vi "Dashboard Main.vi"() -> ()   [LabVIEW 2015]
uses:
  Custom Code/General/RemoteFiles/connectionData.ctl
panel:
  in  "stopButton":bool
  in  "MainDashTab":T1(tab)
  out "Robot IP":string
  in  "Window Docked?":bool
  in  "MainConfigCommunicationData":T3
  out "TeleopImageDisplay":T4(plugin-control)
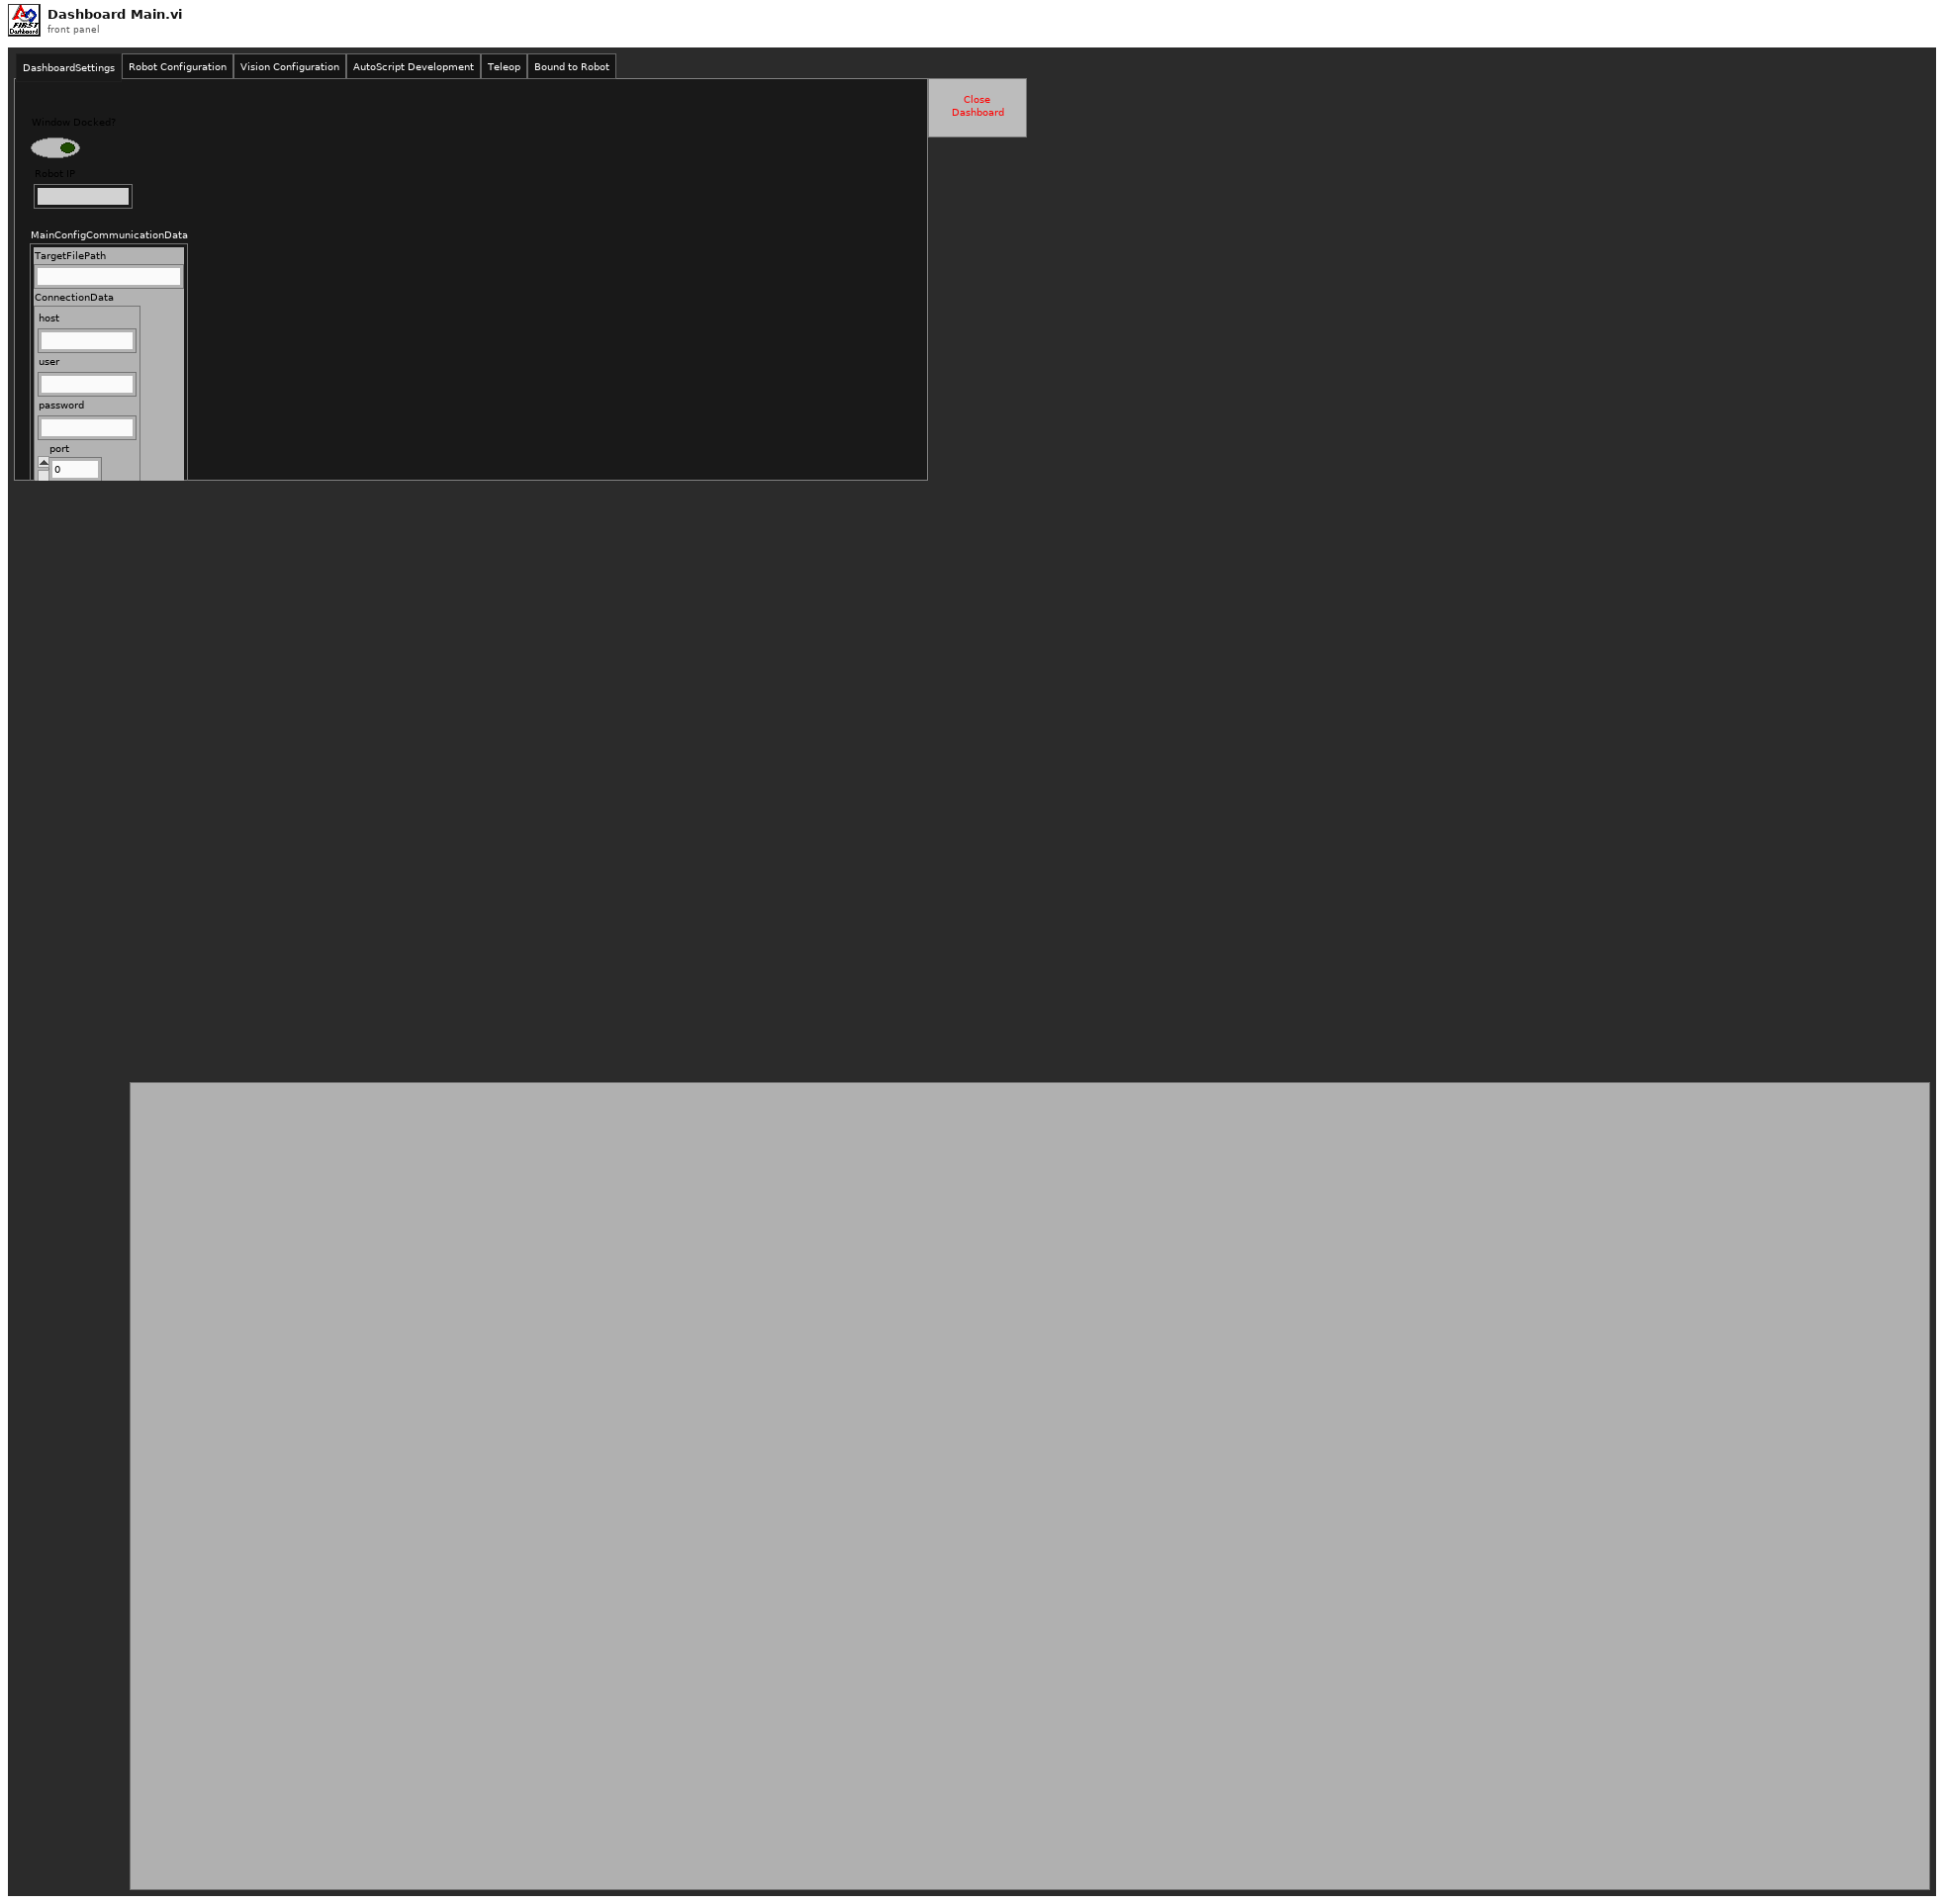
[diagram p1: front panel]
types:
  T1 = enum32{"DashboardSettings", "Robot Configuration", "Vision Configuration", "AutoScript Development", "Teleop", "Bound to Robot"}
  T2 = typedef "connectionData.ctl" = cluster{"host":string, "user":string, "password":string, "port":u16}
  T3 = cluster{"TargetFilePath":string, "ConnectionData":T2}
  T4 = typedef "IMAQ Image.ctl" = refnum<image>
  T5 = cluster{"notifier out":refnum<notifier>, "notifier out":refnum<notifier>, "notifier out":refnum<notifier>}
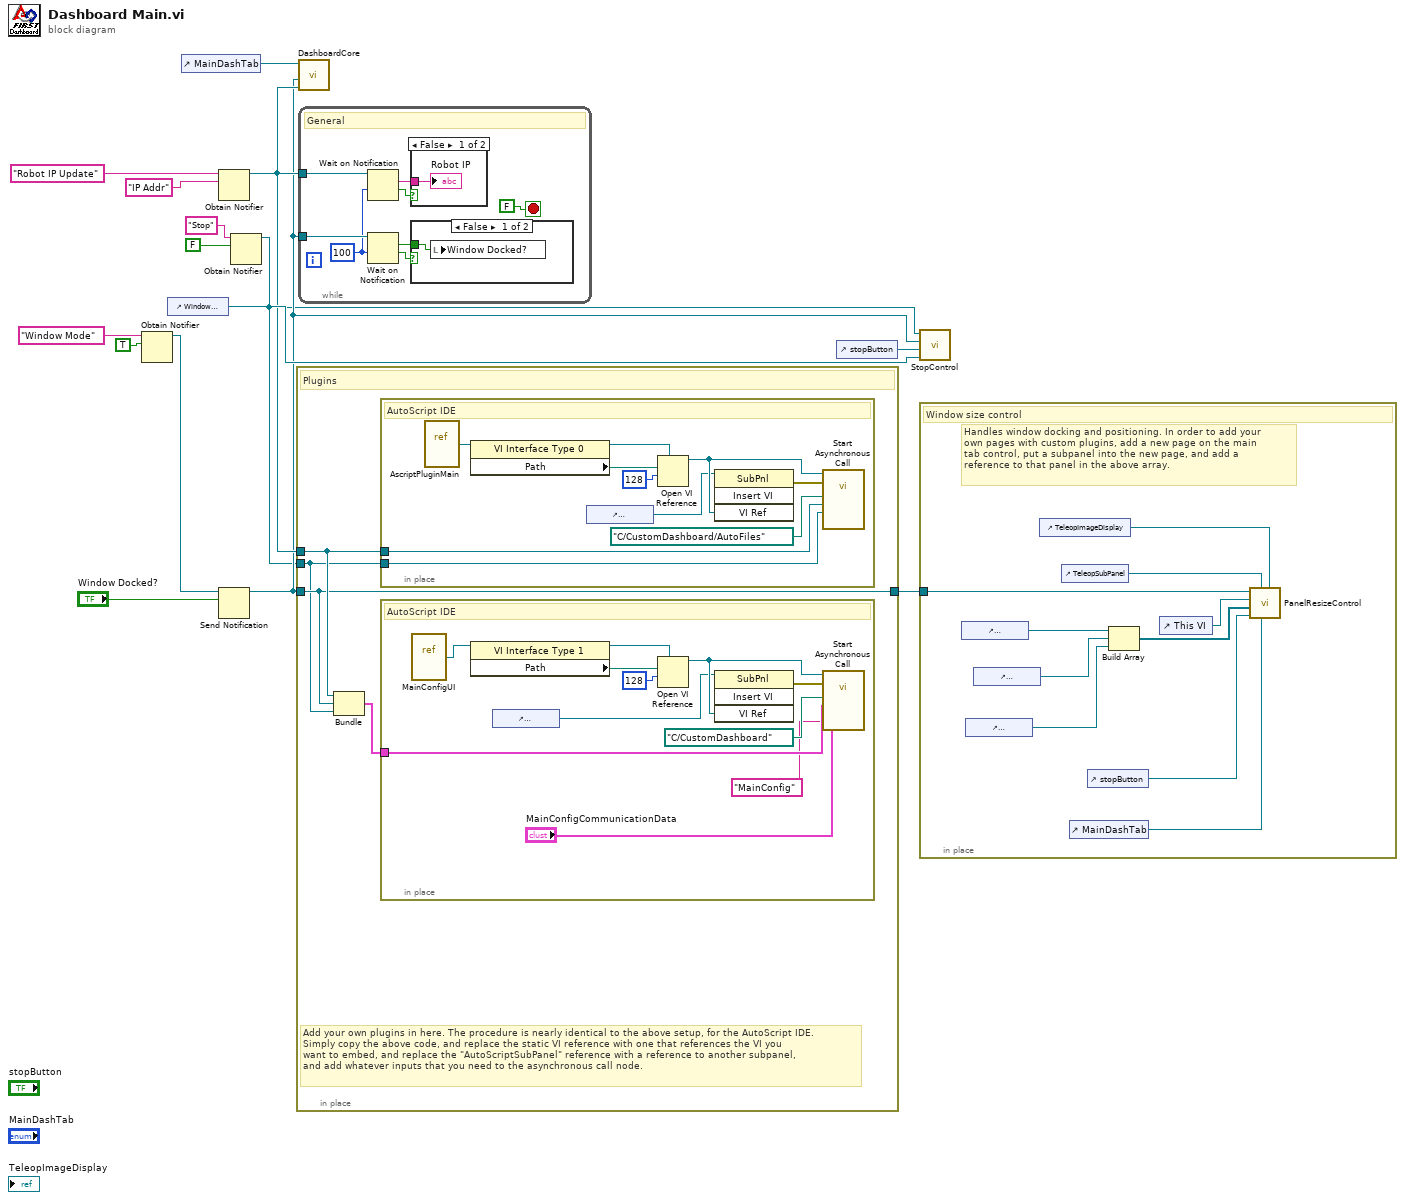
[diagram p0: block diagram]
diagram:
  n1 = Obtain Notifier(name (unnamed)="Window Mode", notification data type=TRUE) -> (notifier out=w5:refnum<notifier>)  [unwired: 2 in, 2 out]
  n2 = control-ref of="Window Docked?"() -> (w7:refnum<vi>)
  n3 = control-ref of="MainDashTab"() -> (w11:refnum<vi>)
  n4 = Obtain Notifier(name (unnamed)="Robot IP Update", notification data type="IP Addr" ("name (unnamed)")) -> (notifier out=w4:refnum<notifier>)  [unwired: 2 in, 2 out]
  n5 = Send Notification(notification="Window Docked?", notifier=w5) -> (notifier out=w3:refnum<notifier>)  [unwired: 1 in, 1 out]
  n6 = Obtain Notifier(name (unnamed)="Stop", notification data type=FALSE) -> (notifier out=w1:refnum<notifier>)  [unwired: 2 in, 2 out]
  n7 = in-place {
    in-place-border: w4 -> [w19]
    in-place-border: w3 -> [w18]
    in-place-border: [w18] -> w2
    in-place-border: w1 -> [w17]
    # "Add your own plugins in here. The procedure is nearly identical to the above setup, for the AutoScript IDE.\nSimply copy the above code, and replace the static VI reference with one that references the VI you\nwant to embed, and replace the \"AutoScriptSubPanel\" reference with a reference to another subpanel,\nand add whatever inputs that you need to the asynchronous call node."
    # "Plugins"
    n8 = Bundle("notifier out"=w19, "notifier out"=w18, "notifier out"=w17) -> (w16:T5)  [unwired: 1 in]
    n9 = in-place {
      in-place-border: w19 -> [w37]
      in-place-border: w17 -> [w31]
      # "AutoScript IDE"
      n10 = vi-ref "AscriptPluginMain.vi"() -> (w36:refnum<vi>)
      n11 = property class="VI Interface Type 0"(reference=w36) -> (reference out=w34:refnum<vi>, "Path"=w35:path)  [unwired: 1 in, 1 out]
      n12 = control-ref of="AutoScriptSubPanel"() -> (w33:refnum<vi>)
      n13 = Open VI Reference(type specifier VI Refnum (for type only)=w34, vi path=w35, options=128) -> (vi reference=w40:refnum<vi>)  [unwired: 3 in, 1 out]
      n14 = invoke class="SubPnl" method="Insert VI"(reference=w33, "VI Ref"=w40) -> (error out=w39:errorcluster)  [unwired: 2 in, 3 out]
      n15 = call-by-ref "Start Asynchronous Call"(reference=w40, error in=w39, "StopNotifier"=w31, "IPnotifier"=w37, "BasePath"=path "C:/CustomDashboard/AutoFiles") -> ()  [unwired: 9 in, 2 out]
    }
    n16 = in-place {
      in-place-border: w16 -> [w23]
      # "AutoScript IDE"
      n17 = vi-ref "MainConfigUI.vi"() -> (w20:refnum<vi>)
      n18 = property class="VI Interface Type 1"(reference=w20) -> (reference out=w26:refnum<vi>, "Path"=w27:path)  [unwired: 1 in, 1 out]
      n19 = control-ref of="MainConfigSubPanel"() -> (w24:refnum<vi>)
      n20 = Open VI Reference(type specifier VI Refnum (for type only)=w26, vi path=w27, options=128) -> (vi reference=w30:refnum<vi>)  [unwired: 3 in, 1 out]
      n21 = invoke class="SubPnl" method="Insert VI"(reference=w24, "VI Ref"=w30) -> (error out=w29:errorcluster)  [unwired: 2 in, 3 out]
      n22 = call-by-ref "Start Asynchronous Call"(reference=w30, error in=w29, "ConfigWindowName"="MainConfig", "Communication Data"="MainConfigCommunicationData", "Notifiers"=w23, "BaseDashPath"=path "C:/CustomDashboard" ("BasePath")) -> ()  [unwired: 8 in, 2 out]
    }
  }
  n23 = call "DashboardCore.vi"("Robot IP notifier in"=w4, "Window mode notifier in"=w3, "Main Dashboard tab"=w11) -> ()  [unwired: 9 in]
  n24 = while {
    tunnel: w4 -> [w47]
    tunnel: w3 -> [w44]
    stop <- FALSE stop-if-true
    w43 = 100 ("timeout in ms (-1)")
    # "General"
    n25 = Wait on Notification(notifier=w47, timeout in ms (-1)=w43) -> (notification=w45:string, timed out?=w46:bool)  [unwired: 2 in, 2 out]
    n26 = Wait on Notification(notifier=w44, timeout in ms (-1)=w43) -> (notification=w41:bool, timed out?=w42:bool)  [unwired: 2 in, 2 out]
    n27 = case shown="False" w46 {
      tunnel: w45 -> [w50 _]
      frame False {
        "Robot IP" <- w50
      }
      frame True {
      }
    }
    n28 = case shown="False" w42 {
      tunnel: w41 -> [w49 _]
      frame False {
        n29 = local write "Window Docked?"(w49) -> ()
      }
      frame True {
      }
    }
  }
  n30 = control-ref of="stopButton"() -> (w8:refnum<vi>)
  n31 = call "StopControl.vi"("WindowButton"=w7, "StopButton"=w8, "Window mode notifier in"=w3, "Stop Notifier in"=w1) -> ()  [unwired: 8 in]
  n32 = in-place {
    in-place-border: w2 -> [w51]
    # "Handles window docking and positioning. In order to add your\nown pages with custom plugins, add a new page on the main\ntab control, put a subpanel into the new page, and add a\nreference to that panel in the above array."
    # "Window size control"
    n33 = control-ref of="VisionConfigSubPanel"() -> (w60:refnum<vi>)
    n34 = control-ref of="MainConfigSubPanel"() -> (w58:refnum<vi>)
    n35 = control-ref of="AutoScriptSubPanel"() -> (w59:refnum<vi>)
    n36 = control-ref of="TeleopImageDisplay"() -> (w52:refnum<vi>)
    n37 = control-ref of="TeleopSubPanel"() -> (w53:refnum<vi>)
    n38 = control-ref of="MainDashTab"() -> (w56:refnum<vi>)
    n39 = control-ref of="stopButton"() -> (w57:refnum<vi>)
    n40 = Build Array(w60, w59, w58) -> (w55:refnum<vi>[])
    n41 = control-ref of="This VI"() -> (w54:refnum<vi>)
    n42 = call "PanelResizeControl.vi"("TeleopDisplay"=w52, "MainDashTab"=w56, "TeleopSubPanel"=w53, "stopButton"=w57, "SubPanels"=w55, "TopLevelVI"=w54, "Window Mode Notifier in"=w51) -> ()  [unwired: 5 in]
  }
